vi "svx_Translate Lines.vi"(5 "Y Offset Per spectrum":dbl[](array[numeric]), 7 "Xoffset per spectrum":dbl[](array[numeric]), 11 "Lines":T1[](array[typedef])) -> (3 "Lines XY Plots":cluster{"X":dbl[], "Y":dbl[]}[](array[cluster]))   [LabVIEW 2017, in "SVX Waterfall Graph.xctl"]
uses:
  <vilib>/addons/_XControls/Waterfall Graph/SVX Waterfall Graph.xctl
  <vilib>/addons/_NISVFA/_Shared subVIs/Controls/svc_Cluster of Array of Cluster of XYZ.ctl
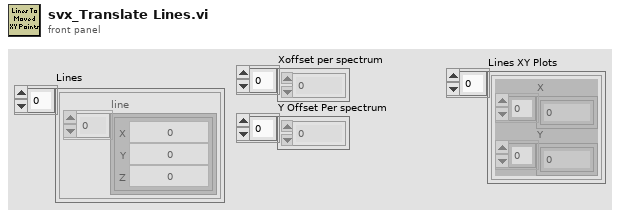
[diagram p1: front panel]
types:
  T1 = typedef "svc_Cluster of Array of Cluster of XYZ.ctl" = cluster{"line":cluster{"X":dbl, "Y":dbl, "Z":dbl}[]}
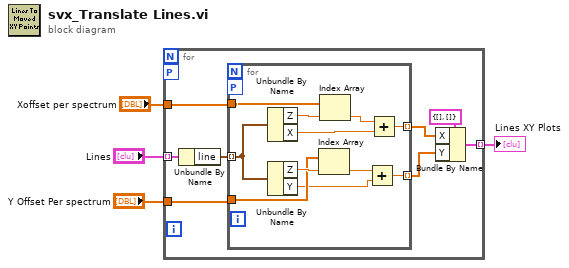
[diagram p0: block diagram]
diagram:
  n1 = for {
    tunnel: "Lines" -> [w10] mode=indexing
    tunnel: "Xoffset per spectrum" -> [w12]
    tunnel: "Y Offset Per spectrum" -> [w11]
    tunnel: [w5] -> w1 mode=indexing
    workers-P: _ -> [_]
    n2 = Unbundle By Name(w10) -> ("line"=w9:cluster{"X":dbl, "Y":dbl, "Z":dbl}[])
    n3 = for {
      tunnel: w9 -> [w18] mode=indexing
      tunnel: w12 -> [w15]
      tunnel: w11 -> [w16]
      tunnel: [w23] -> w7 mode=indexing
      tunnel: [w22] -> w6 mode=indexing
      workers-P: _ -> [_]
      n4 = Unbundle By Name(w18) -> ("Z"=w17:dbl, "X"=w14:dbl)
      n5 = Unbundle By Name(w18) -> ("Z"=w21:dbl, "Y"=w13:dbl)
      n6 = Index Array(array=w16, index=w21) -> (element=w19:dbl)
      n7 = Index Array(array=w15, index=w17) -> (element=w20:dbl)
      n8 = Add(x=w19, y=w13) -> (x+y=w22:dbl)
      n9 = Add(x=w20, y=w14) -> (x+y=w23:dbl)
    }
    n10 = Bundle By Name(cluster=cluster{"X":dbl[], "Y":dbl[]} {"X"=[], "Y"=[]}, "X"=w7, "Y"=w6) -> (w5:cluster{"X":dbl[], "Y":dbl[]})
  }
  "Lines XY Plots" <- w1
